vi "RT_CreateRTNetworkStreamReader.vi"(8 "ErrorIn":errorcluster, 11 "RT Stream Name":string="Mast/Trig") -> (0 "ErrorOut":errorcluster, 3 "UI Stream Name":refnum<k21>)   [LabVIEW 2018]
uses:
  Controls/Clusts/StreamClust.ctl
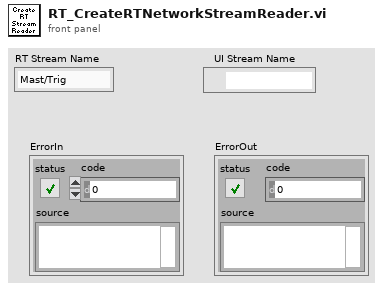
[diagram p1: front panel]
types:
  T1 = typedef "StreamClust.ctl" = cluster{u16, variant}
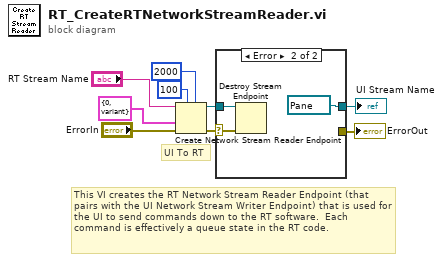
[diagram p0: block diagram]
diagram:
  # "This VI creates the RT Network Stream Reader Endpoint (that pairs with the UI Network Stream Writer Endpoint) that is used for the UI to send commands down to the RT software.  Each command is effectively a queue state in the RT code."
  # "UI To RT"
  n1 = Create Network Stream Reader Endpoint(5:2000 ("Network Stream Connect Timeout (ms)"), 7:100 ("reader buffer size"), 8:"ErrorIn", 9:T1 {0, variant}, 11:"RT Stream Name") -> (0:w8:errorcluster, 3:w2:refnum<k21>)  [unwired: 2 in]
  n2 = case shown="Error" w8 {
    selector: w8 -> [w11 w14]
    tunnel: [w11 _] -> w9
    tunnel: w2 -> [w10 w13]
    tunnel: [w10 refnum<k21> refnum ("reader endpoint")] -> w1
    frame No Error {
    }
    frame Error {
      n3 = Destroy Stream Endpoint(8:w14, 11:w13) -> ()  [unwired: 1 out]
    }
  }
  "ErrorOut" <- w9
  "UI Stream Name" <- w1
